vi "Grab Image.vi"() -> ()   [LabVIEW 2014]
uses:
  4.Other/header ctl/Offset.ctl
  4.Other/header ctl/file number.ctl
  <vilib>/vision/Image Controls.llb/IMAQ Image.ctl
  <vilib>/userdefined/High Color/IMAQdx.ctl
  4.Other/header ctl/Header file data.ctl
  4.Other/header ctl/Offset table.ctl
  <vilib>/Analysis/baseanly.llb/Mean (DBL).vi
  <vilib>/vision/driver/NI_Vision_Acquisition_Software.lvlib
  <resource>/objmgr/imaqdx.rc
  <vilib>/vision/NI_Vision_Development_Module.lvlib
  <vilib>/Analysis/NI_AALBase.lvlib
panel:
  in  "Reset BM":bool
  out "error out":errorcluster
  out "Global Rectangle":i32[](array[numeric])
  out "BMy array":dbl[](array[numeric])
  out "BMx array":dbl[](array[numeric])
  out "y array":dbl[](array[numeric])
  out "x array":dbl[](array[numeric])
  in  "AutoGain":enum16{"None", "Auto Once", "Continuous"}(ring)
  out "mean fps":dbl format="%0.2f"
  in  "Array":string[](array[string])=["BMx (nm)", "BMy (nm)", "xy ratio"]
  out "Results":dbl[](array[numeric])
  out "Saved Frame":u32
  out "acquire time array (ms)":u32[](array[numeric])
  in  "Extract bead?":bool
  out "frame acquired":i32
  out "Offset array":cluster{"offset":T1, "file number":T2}[](array[cluster])
  out "resized TTB":u32[](array[numeric])
  out "True acquired frame":u32
  in  "wait time between \neach grab (ms)":u32=30
  out "fps (Hz)":dbl
  out "TTB array (ms)\ntime axis (ms)":u32[](array[numeric])
  out "Glimpse refnum Array":refnum<file>[](array[refnum])
  in  "T = Stop Record":bool
  in  "T = Record Sequence":bool
  out "Finish Save?":bool
  out "Pixel depth":i16
  out "Path String Array":string[](array[string])
  in  "Tab Control":T3(tab)
  in  "Set Record Frame#":u32=30000
  out "Width":i32
  out "Height":i32
  in  "Data type":enum16{"U8", "I16"}(ring)
  in  "Select a Folder":path
  out "size of one frame (byte)":u32
  out "Frame# of one .Glimpse \n(2Gb)":u32
  out "Estimated total file size (byte, b)":u32
  out "Estimated total file size (Kb)":dbl
  out "image in Queue":i32(slide) min=0 max=180 step=30 scale=0.18..200.0
  out "pixel# of a image":i32
  out "Estimated a file size (byte, b)":u32
  out "Write to file num":u32
  out "avg. fps for recording (Hz)":dbl
  in  "Set Height":dbl=630.0
  in  "Set Width":dbl=1120.0
  in  "T = Auto-Set Exposure\nF = Manual":bool=TRUE
  in  "Manual Set\nExposure Time (ms)":dbl=30.0
  out "Image Display":T4(plugin-control)
  out "Image Extracted":T4(plugin-control)
  # "1120"
  # "width : max 1920"
  # "height max : 1200"
  # "630"
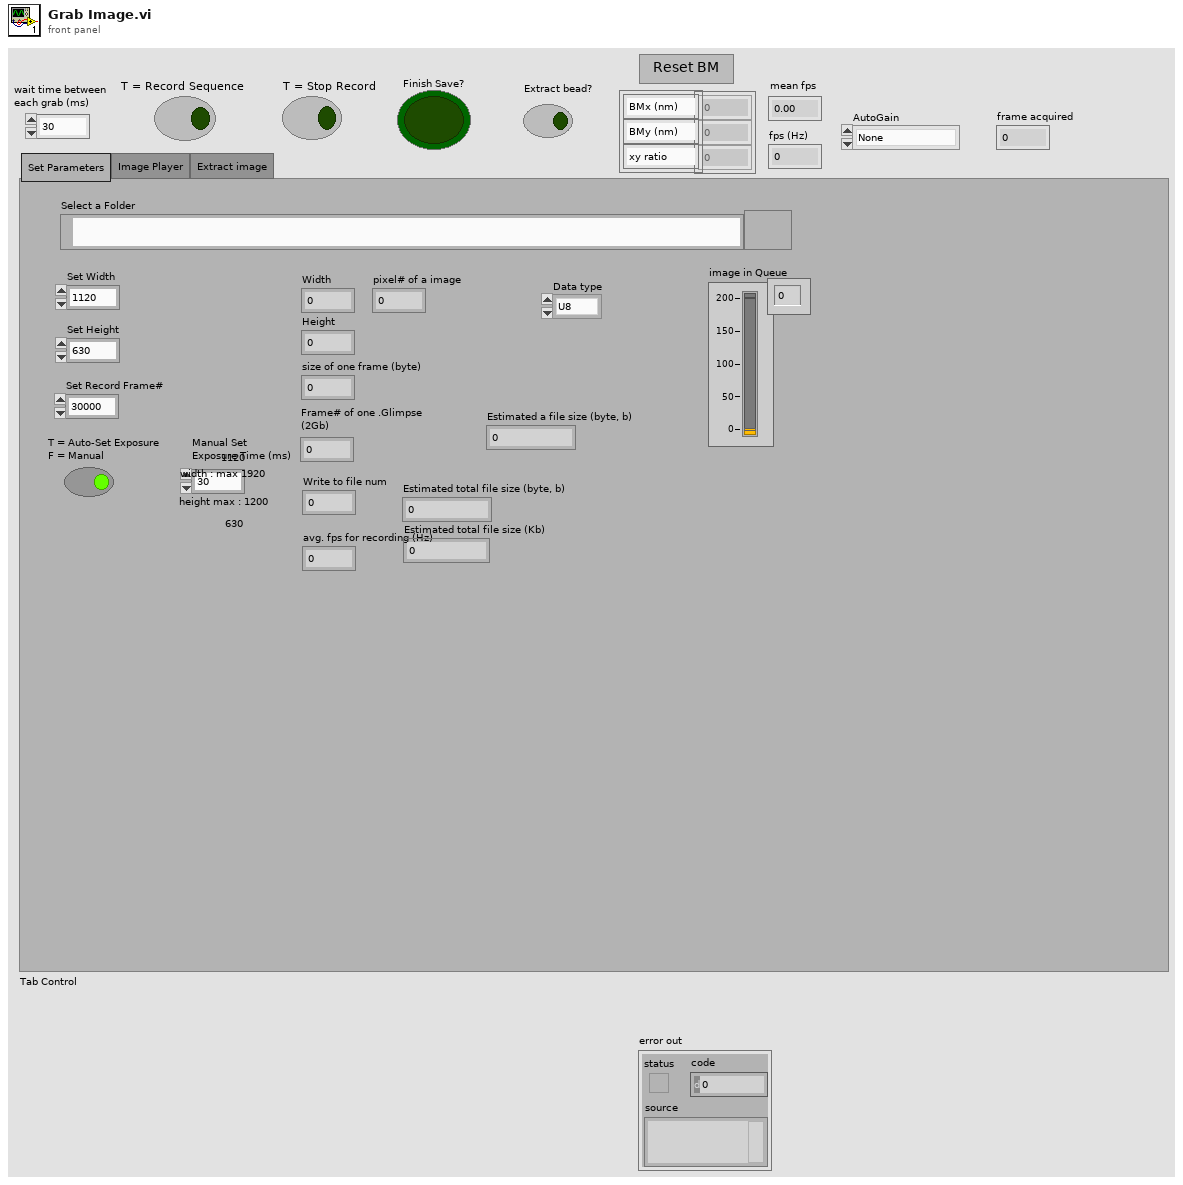
[diagram p1: front panel]
types:
  T1 = typedef "Offset.ctl" = i32
  T2 = typedef "file number.ctl" = u8
  T3 = enum32{"Set Parameters", "Image Player", "Extract image"}
  T4 = typedef "IMAQ Image.ctl" = refnum<image>
  T5 = typedef "IMAQdx.ctl" = refnum<k21>
  T6 = typedef "Image Type" = u32
  T7 = cluster{"Grab Image":T4, "max queue size (-1, unlimited)":u32}
  T8 = cluster{"Global Rectangle":i32[], "Contours":cluster{"Contour Type":u32, "ROI Type":u32, "Points":i32[]}[]}
  T9 = enum16{"open", "replace", "create", "open or create", "replace or create", "replace or create with confirmation"}
  T10 = typedef "Header file data.ctl" = cluster{"Frames Acquired":u32, "Region width":i32, "Region height":i32, "Element 0 of TTB":u32, "time of 1st frame, \nsec since 1/1/04":dbl, "TTB Array (ms)":u32[], "Offsets Array":T11, "Pixel depth":u32}
  T11 = typedef "Offset table.ctl" = cluster{"offset":T1, "file number":T2}[]
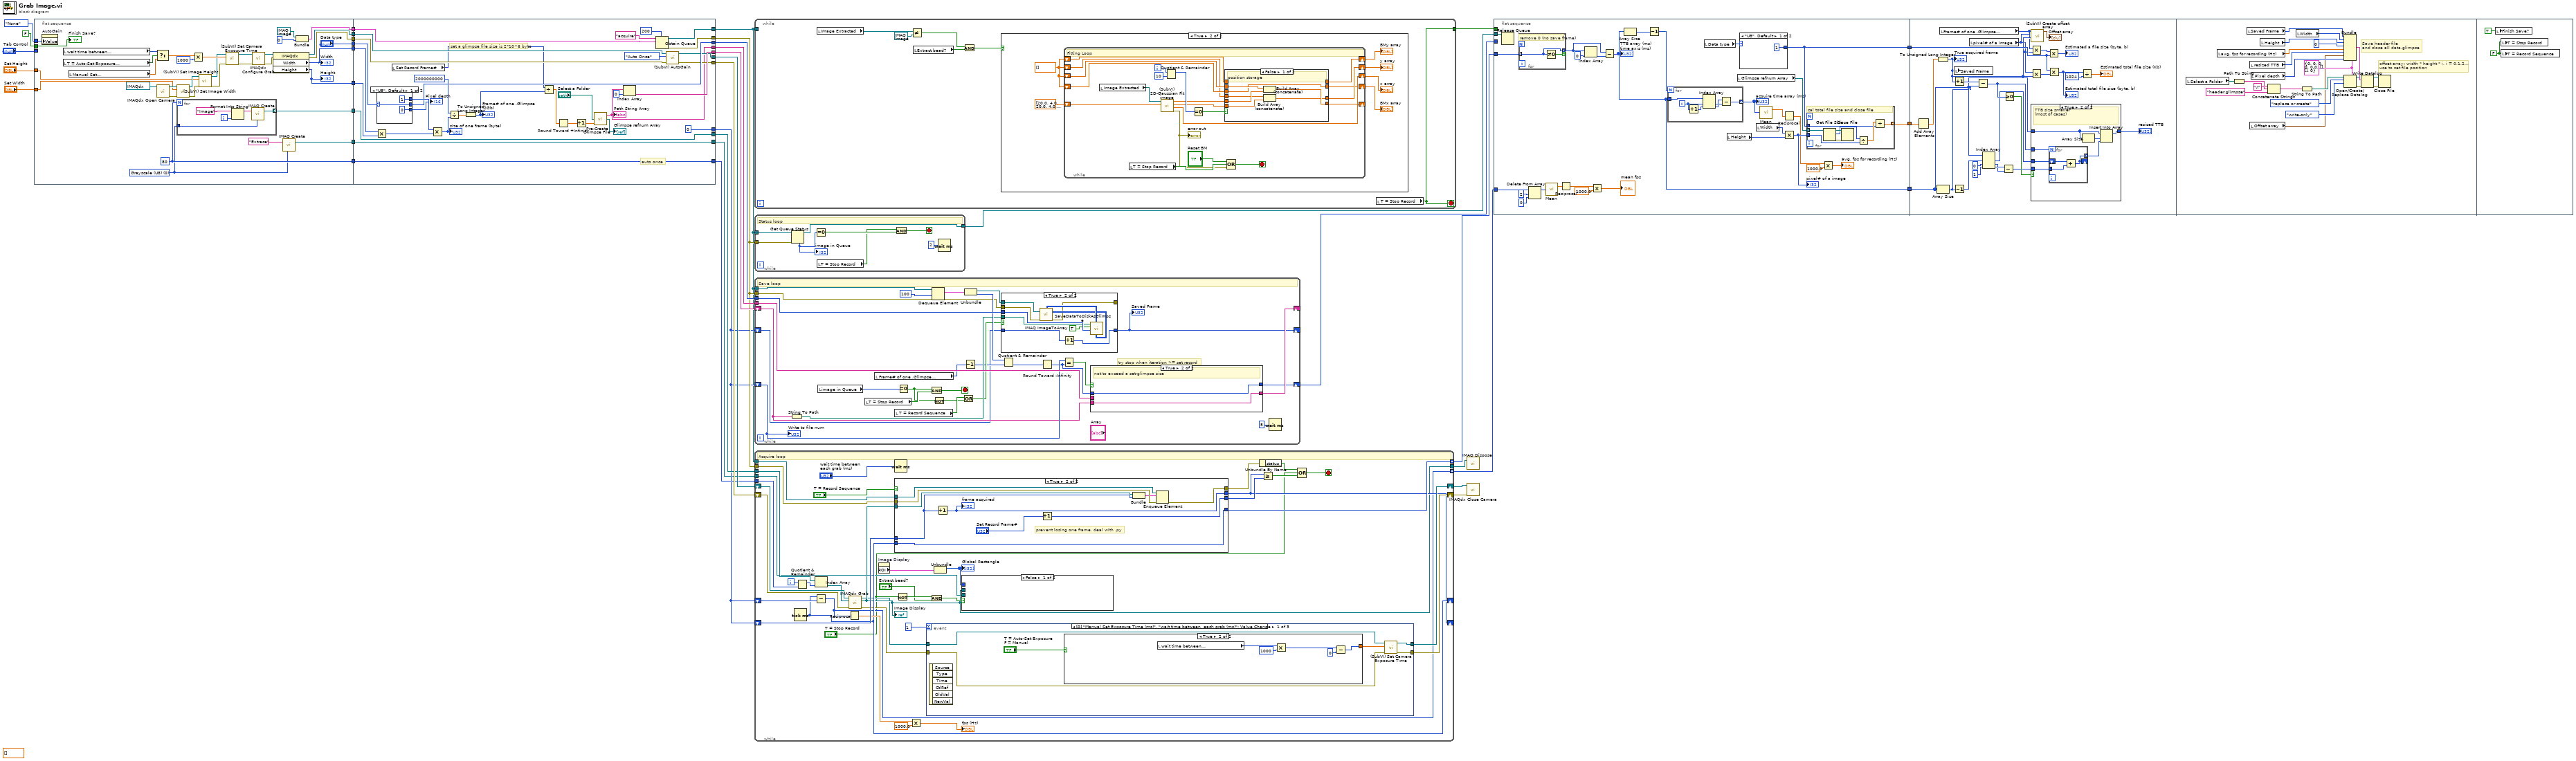
[diagram p0: block diagram]
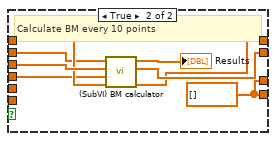
[diagram p3: hidden frame]
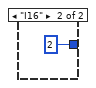
[diagram p4: hidden frame]
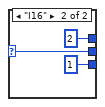
[diagram p6: hidden frame]
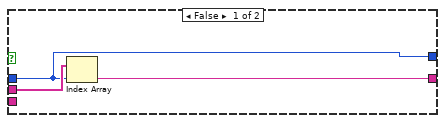
[diagram p8: hidden frame]
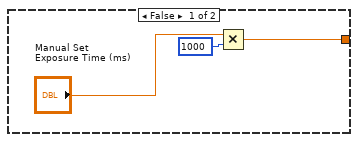
[diagram p9: hidden frame]
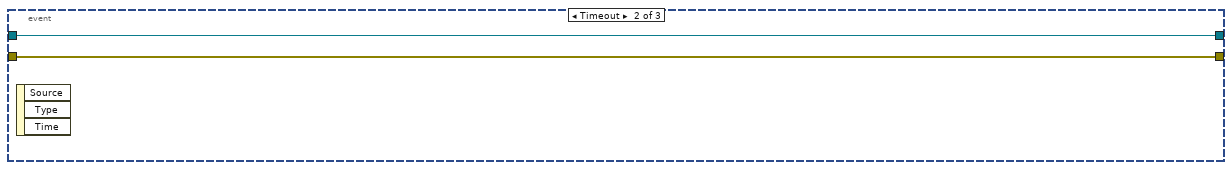
[diagram p10: hidden frame]
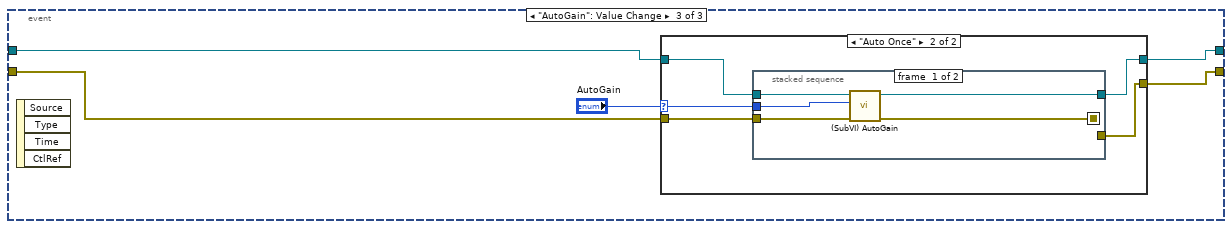
[diagram p11: hidden frame]
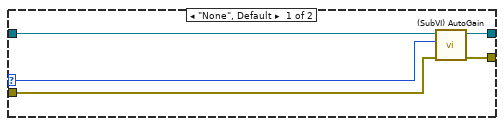
[diagram p12: hidden frame]
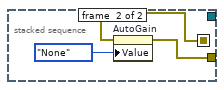
[diagram p13: hidden frame]
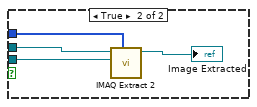
[diagram p14: hidden frame]
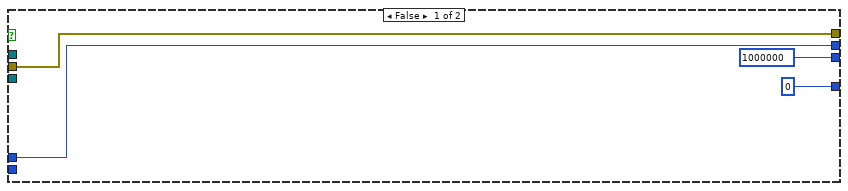
[diagram p15: hidden frame]
diagram:
  (unwired) dbl[] []
  n1 = flat-sequence {
    tunnel: [w61] -> w33
    tunnel: [w60] -> w32
    tunnel: [w70] -> w29
    tunnel: [w69] -> w28
    tunnel: ["Data type"] -> w26
    tunnel: [w65] -> w24
    tunnel: [w59] -> w21
    tunnel: [w58] -> w19
    tunnel: "Tab Control" -> [_]
    tunnel: FALSE ("Finish Save?") -> [w57]
    tunnel: "Set Width" -> [w43]
    tunnel: "Set Height" -> [w42]
    tunnel: [w54] -> w6
    tunnel: enum16{"None", "Auto Once", "Continuous"}."None" ("AutoGain") -> [w41]
    tunnel: [w88] -> w30
    tunnel: w33 -> [w90]
    tunnel: [w87] -> w31
    tunnel: w32 -> [w89]
    tunnel: w29 -> [w109]
    tunnel: w28 -> [w108]
    tunnel: w26 -> [w102]
    tunnel: [w101] -> w25
    tunnel: w24 -> [w95]
    tunnel: [w100] -> w20
    tunnel: w21 -> [w100]
    tunnel: [w99] -> w18
    tunnel: w19 -> [w99]
    tunnel: [w85] -> w16
    tunnel: [0] -> w10
    tunnel: [w96] -> w12
    tunnel: [w94] -> w2
    tunnel: [w93] -> w11
    tunnel: w6 -> [w77]
    tunnel: [w77] -> w5
    frame #0 {
      w58 = 80 ("# Of Buffers")
      w55 = T6 0 items=["Grayscale (U8)", "Grayscale (I16)", "Grayscale (SGL)", "Complex (CSG)", "RGB (U32)", "HSL (U32)", "RGB (U64)", "Grayscale (U16)"] ("Image Type")
      n2 = property on="AutoGain" class="Enum (strict)"("Value"=w41) -> ()  [unwired: 2 in, 2 out]
      n3 = local read "wait time between \neach grab (ms)"() -> (w38:u32)
      n4 = local read "T = Auto-Set Exposure\nF = Manual"() -> (w40:bool)
      n5 = local read "Manual Set\nExposure Time (ms)"() -> (w39:dbl)
      n6 = Select(t=w38, s=w40, f=w39) -> (s? t:f=w37:dbl)
      n7 = call <vilib>:"IMAQdx Open Camera.vi"("Session In"=T5 "cam2") -> ("error out"=w44:errorcluster, "Session Out"=w49:T5)  [unwired: 9 in]
      n8 = call "(SubVI) Set Image Width.vi"("error in (no error)"=w44, "Set Width"=w43, "Refnum in"=w49) -> ("error out"=w45:errorcluster, "Refnum out"=w48:T5)  [unwired: 7 in]
      n9 = for {
        N: w58 -> [_]
        tunnel: [w75] -> w59 mode=indexing
        tunnel: w55 -> [w71]
        i -> [w74]
        n10 = Format Into String(initial string="Image" ("Image Name"), w74) -> (resulting string=w72:string)  [unwired: 2 in, 1 out]
        n11 = call "IMAQ Create"("Image Name"=w72, "Image Type"=w71) -> ("New Image"=w75:T4)  [unwired: 3 in, 1 out]
      }
      n12 = Multiply(x=w37, y=u32 1000) -> (x*y=w50:dbl)
      n13 = call "(SubVI) Set Image Height.vi"("error in (no error)"=w45, "Set Height"=w42, "Refnum in"=w48) -> ("error out"=w46:errorcluster, "Refnum out"=w47:T5)  [unwired: 7 in]
      n14 = call "(SubVI) Set Camera Exposure Time.vi"("error in (no error)"=w46, "ExposureTime (us)"=w50, "Refnum in"=w47) -> ("error out"=w53:errorcluster, "Refnum out"=w52:T5)  [unwired: 7 in]
      n15 = call <vilib>:"IMAQdx Configure Grab.vi"("error in"=w53, "Session In"=w52) -> ("error out"=w62:errorcluster, "Session Out"=w63:T5)  [unwired: 8 out]
      n16 = property class="IMAQdx"(reference=w63, error in=w62) -> (reference out=w61:T5, error out=w60:errorcluster, "Width"=w70:u32, "Height"=w69:u32)
      "Width" <- w70
      "Height" <- w69
      n17 = call "IMAQ Create"("Image Name"="Extrace", "Image Type"=w55) -> ("New Image"=w54:T4)  [unwired: 3 in, 1 out]
      n18 = Bundle("Grab Image"=T4 refnum, "max queue size (-1, unlimited)"=u32 0) -> (w65:T7)  [unwired: 1 in]
      "Finish Save?" <- w57
    }
    frame #1 {
      # "auto once"
      # "set a glimpse file size is 2*10^6 byte"
      n19 = Multiply(x=w109, y=w108) -> (x*y=w107:u32)
      n20 = case shown="\"U8\", Default" w102 {
        selector: w102 -> [w111 w114]
        tunnel: [1 2] -> w106
        tunnel: [w111 w114] -> w101
        tunnel: [i16 0 i16 1] -> w91
        frame "U8", Default {
        }
        frame "I16" {
        }
      }
      "Pixel depth" <- w91
      n21 = local read "Set Record Frame#"() -> (w83:u32)
      n22 = Multiply(x=w106, y=w107) -> (x*y=w104:u32)
      "size of one frame (byte)" <- w104
      n23 = Divide(x=2000000000, y=w104) -> (x/y=w103:dbl)
      n24 = To Unsigned Long Integer(number=w103) -> (unsigned 32bit integer=w82:u32)
      "Frame# of one .Glimpse \n(2Gb)" <- w82
      n25 = Divide(x=w83, y=w82) -> (x/y=w81:dbl)
      n26 = Round Toward +Infinity(x=w81) -> (ceil(x): smallest int >= x=w80:dbl)
      n27 = Increment(x=w80) -> (x+1=w79:dbl)
      n28 = call "Pre-Create Glimpse File.vi"("pre-created file #"=w79, "Select a Folder"="Select a Folder") -> ("refnum Array"=→"Glimpse refnum Array":refnum<file>[], "Path String Array"=w85:string[])  [unwired: 2 in]
      "Path String Array" <- w85
      n29 = Index Array(array=w85, index=0) -> (element=w96:string)
      n30 = Obtain Queue(max queue size (-1, unlimited)=200, name (unnamed)="acquire", element data type=w95) -> (queue out=w94:refnum<queue>, error out=w93:errorcluster)  [unwired: 2 in, 1 out]
      n31 = call "(SubVI) AutoGain.vi"("error in (no error)"=w89, "AutoMode"=enum16{"None", "Auto Once", "Continuous"}."Auto Once", "Refnum in"=w90) -> ("error out"=w87:errorcluster, "Refnum out"=w88:T5)  [unwired: 7 in]
    }
  }
  n32 = while {
    tunnel: w2 -> [_]
    tunnel: [w119] -> w1
    stop <- w119 stop-if-true
    n33 = local read "Image Extracted"() -> (w121:T4)
    n34 = Not Equal?(x=w121, y=T4 refnum ("Grab Image")) -> (x != y?=w118:bool)
    n35 = local read "Extract bead?"() -> (w117:bool)
    n36 = And(x=w118, y=w117) -> (x .and. y?=w116:bool)
    n37 = case shown="True" w116 {
      frame False {
      }
      frame True {
        w127 = dbl[] []
        n38 = while {
          shift-right: [w133] -> w126
          shift-left: w127 -> [w142]
          shift-right: [w132] -> w125
          shift-left: w127 -> [w141]
          shift-right: [w134] -> w124
          shift-left: w127 -> [w140]
          shift-right: [w135] -> w123
          shift-left: w127 -> [w139]
          shift-right: [w138] -> _
          shift-left: dbl[] [20.0, 4.0, 20.0, 4.0, 40.0, 127.0] ("initial parameters") -> [w137]
          i -> [w143]
          stop <- w128 stop-if-true
          # "Fitting Loop"
          n39 = local read "Image Extracted"() -> (w136:T4)
          n40 = local read "T = Stop Record"() -> (w130:bool)
          n41 = call "(SubVI) 2D-Gaussian Fit image.vi"("initial parameters"=w137, "Input Image"=w136) -> ("error out"=w129:errorcluster, "best fit parameters"=w138:dbl[], "y position (nm)"=w145:dbl, "x position (nm)"=w146:dbl)  [unwired: 6 in]
          "error out" <- w129
          n42 = Quotient & Remainder(x=w143, y=10) -> (x-y*floor(x/y)=w147:i32)  [unwired: 1 out]
          n43 = Equal To 0?(x=w147) -> (x = 0?=w144:bool)
          n44 = case shown="False" w144 {
            tunnel: w142 -> [w153 w159]
            tunnel: w140 -> [w152 w158]
            tunnel: [w154 w160] -> w133
            tunnel: [w151 w160] -> w134
            tunnel: [w150 w164] -> w132
            tunnel: [w149 w163] -> w135
            tunnel: w141 -> [w150 w162]
            tunnel: w139 -> [w149 w161]
            tunnel: w146 -> [w156 _]
            tunnel: w145 -> [w155 _]
            frame False {
              # "position storage"
              n45 = Build Array (concatenate)(w153, w156) -> (w154:dbl[])
              n46 = Build Array (concatenate)(w152, w155) -> (w151:dbl[])
            }
            frame True {
              w160 = dbl[] []
              # "Calculate BM every 10 points"
              n47 = call "(SubVI) BM calculator.vi"("BMy array in (nm)"=w161, "y position array in (nm)"=w158, "BMx array in (nm)"=w162, "x position array in (nm)"=w159) -> ("BMy array appended (nm)"=w163:dbl[], "BMx array appended (nm)"=w164:dbl[], "Results"=→"Results":dbl[])  [unwired: 1 in]
            }
          }
          n48 = Compound Arithmetic op=OR("Reset BM", w130, w129) -> (w128:bool)
        }
        "x array" <- w126
        "y array" <- w124
        "BMx array" <- w125
        "BMy array" <- w123
      }
    }
    n49 = local read "T = Stop Record"() -> (w119:bool)
  }
  n50 = while {
    tunnel: w2 -> [w172]
    tunnel: [w171] -> w22
    tunnel: w11 -> [w170]
    stop <- w165 stop-if-true
    # "Status loop"
    n51 = Get Queue Status(queue=w172, error in (no error)=w170) -> (queue out=w171:refnum<queue>, # elements in queue=w168:i32)  [unwired: 1 in, 6 out]
    "image in Queue" <- w168
    n52 = Equal To 0?(x=w168) -> (x = 0?=w169:bool)
    n53 = local read "T = Stop Record"() -> (w166:bool)
    n54 = And(x=w166, y=w169) -> (x .and. y?=w165:bool)
    n55 = Wait (ms)(milliseconds to wait=u32 2) -> ()  [unwired: 1 out]
  }
  n56 = while {
    tunnel: w2 -> [w201]
    tunnel: w11 -> [w200]
    tunnel: w25 -> [w199]
    shift-right: [w188] -> w23
    shift-left: w10 -> [w193]
    shift-right: [w192] -> _
    shift-left: w12 -> [w190]
    tunnel: w16 -> [w194]
    shift-right: [w173] -> _
    shift-left: w10 -> [w174]
    stop <- w177 stop-if-true
    # "try stop when iteration >= set record"
    # "Save loop"
    n57 = String To Path(string=w190) -> (path=w191:path)
    n58 = local read "image in Queue"() -> (w183:i32)
    n59 = local read "T = Stop Record"() -> (w185:bool)
    n60 = local read "Frame# of one .Glimpse \n(2Gb)"() -> (w175:u32)
    n61 = local read "T = Record Sequence"() -> (w182:bool)
    n62 = Equal To 0?(x=w183) -> (x = 0?=w180:bool)
    n63 = And(x=w180, y=w185) -> (x .and. y?=w177:bool)
    n64 = Dequeue Element(queue=w201, timeout in ms (-1)=100, error in (no error)=w200) -> (element=w198:T7, error out=w184:errorcluster)  [unwired: 2 out]
    n65 = Not(x=w180) -> (.not. x?=w181:bool)
    n66 = Or(x=w182, y=w181) -> (x .or. y?=w179:bool)
    n67 = Decrement(x=w175) -> (x-1=w176:u32)
    n68 = Unbundle(w198) -> ("Grab Image"=w187:T4, "max queue size (-1, unlimited)"=w197:u32)
    n69 = case shown="True" w179 {
      tunnel: w199 -> [_ w213]
      tunnel: w191 -> [_ w212]
      tunnel: w187 -> [_ w208]
      tunnel: w184 -> [w203 w207]
      tunnel: [w203 w206] -> _
      tunnel: w174 -> [w202 w205]
      tunnel: [w202 w204] -> w173
      frame False {
      }
      frame True {
        n70 = call "IMAQ ImageToArray"("error in (no error)"=w207, "Image"=w208) -> ("error out"=w206:errorcluster, "Image Pixels (U8)"=w210:u8[][], "Image Pixels (I16)"=w209:i16[][])  [unwired: 2 in, 2 out]
        n71 = Increment(x=w205) -> (x+1=w204:i32)
        n72 = call "SaveDataToDiskAsGlimpse.vi"("Read or Write Path"=w212, "Array (U8)"=w210, "T = AddNewData\nF = if exist, OverWrite or CreateNew"=TRUE ("T = AddNewData\nF = if exist, OverWrite or CreateNew"), "Data type"=w213, "Array (I16)"=w209) -> ()  [unwired: 3 in, 1 out]
      }
    }
    "Saved Frame" <- w173
    n73 = Quotient & Remainder(x=w197, y=w176) -> (floor(x/y)=w196:u32)  [unwired: 1 out]
    n74 = Round Toward -Infinity(1:w196) -> (0:w189:u32)
    n75 = Equal?(x=w193, y=w189) -> (x = y?=w195:bool)
    n76 = case shown="True" w195 {
      tunnel: w194 -> [w216 _]
      tunnel: w189 -> [w214 w217]
      tunnel: [w215 w218] -> w192
      tunnel: w190 -> [_ w218]
      tunnel: [w214 w217] -> w188
      frame False {
        n77 = Index Array(array=w216, index=w214) -> (element=w215:string)
      }
      frame True {
        # "not to exceed a set-glimpse size"
      }
    }
    n78 = Wait (ms)(milliseconds to wait=u32 5) -> ()  [unwired: 1 out]
    "Write to file num" <- w193
  }
  n79 = while {
    tunnel: [w231] -> w34
    tunnel: w2 -> [w253]
    shift-right: [w233] -> _
    shift-left: w10 -> [w249]
    tunnel: w11 -> [w248]
    shift-right: [w235] -> _
    shift-left: w10 -> [w247]
    tunnel: w20 -> [w242]
    tunnel: w18 -> [w240]
    tunnel: [w234] -> w17 mode=indexing
    shift-right: [w236] -> w36
    shift-left: w30 -> [w256]
    shift-right: [w237] -> w35
    shift-left: w31 -> [w255]
    tunnel: w5 -> [w232]
    tunnel: [w226] -> w4 mode=indexing
    i -> [w225]
    stop <- w238 stop-if-true
    # "Acquire loop"
    n80 = Tick Count (ms)() -> (millisecond timer value=w235:u32)
    n81 = Quotient & Remainder(x=w225, y=w240) -> (x-y*floor(x/y)=w243:i32)  [unwired: 1 out]
    n82 = Subtract(x=w235, y=w247) -> (x-y=w226:u32)
    n83 = Index Array(array=w242, index=w243) -> (element=w241:T4)
    n84 = Reciprocal(x=w226) -> (1/x=w246:dbl)
    n85 = call <vilib>:"IMAQdx Grab.vi"("error in"=w255, "Image In"=w241, "Session In"=w256) -> ("error out"=w228:errorcluster, "Image Out"=w231:T4, "Session Out"=w229:T5)  [unwired: 1 in, 5 out]
    "Image Display" <- w231
    n86 = property on="Image Display" class="ImageControl"() -> ("ROI"=w230:T8)  [unwired: 2 in, 2 out]
    n87 = Wait (ms)(milliseconds to wait="wait time between \neach grab (ms)") -> ()  [unwired: 1 out]
    n88 = case shown="True" "T = Record Sequence" {
      tunnel: w253 -> [_ w313]
      tunnel: w231 -> [_ w310]
      tunnel: w248 -> [w303 w312]
      tunnel: [w303 w311] -> w252
      tunnel: w249 -> [w302 w309]
      tunnel: [w302 w308] -> w233
      tunnel: [u32 1000000 ("Set Record Frame#") w304] -> w239
      tunnel: [u32 0 ("millisecond timer value") w306] -> w234
      tunnel: w235 -> [_ w306]
      frame False {
      }
      frame True {
        # "prevent losing one frame, deal with .py"
        n89 = Increment(x=w309) -> (x+1=w308:i32)
        "frame acquired" <- w308
        n90 = Increment(x="Set Record Frame#") -> (x+1=w304:u32)
        n91 = Bundle("Image Out"=w310, w309) -> (w307:cluster{"Image Out":T4, i32})  [unwired: 1 in]
        n92 = Enqueue Element(queue=w313, element=w307, error in (no error)=w312) -> (error out=w311:errorcluster)  [unwired: 1 in, 2 out]
      }
    }
    n93 = Not(x="T = Stop Record") -> (.not. x?=w222:bool)
    n94 = Multiply(x=w246, y=1000.0) -> (x*y=→"fps (Hz)":dbl)
    n95 = event shown="[0] \"Manual Set Exposure Time (ms)\", \"wait time between  each grab (ms)\": Value Change" {
      selector: _ -> [_ _ _]
      dyn-events: _ -> [_ _ _]
      timeout: 1 -> [_ _ _]
      tunnel: w229 -> [w262 w272 w277]
      tunnel: [w261 w272 w275] -> w236
      tunnel: w228 -> [w260 w271 w276]
      tunnel: [w259 w271 w273] -> w237
      event "Manual Set\nExposure Time (ms)", "wait time between \neach grab (ms)": Value Change {
        n96 = event-data() -> ()  [unwired: 1 in, 6 out]
        n97 = case shown="True" "T = Auto-Set Exposure\nF = Manual" {
          tunnel: [w263 w267] -> w257
          frame False {
            n98 = Multiply(x="Manual Set\nExposure Time (ms)", y=u32 1000) -> (x*y=w263:dbl)
          }
          frame True {
            n99 = local read "wait time between \neach grab (ms)"() -> (w266:u32)
            n100 = Multiply(x=w266, y=u32 1000) -> (x*y=w269:u32)
            n101 = Subtract(x=w269, y=u32 0) -> (x-y=w267:u32)
          }
        }
        n102 = call "(SubVI) Set Camera Exposure Time.vi"("error in (no error)"=w260, "ExposureTime (us)"=w257, "Refnum in"=w262) -> ("error out"=w259:errorcluster, "Refnum out"=w261:T5)  [unwired: 7 in]
      }
      event Timeout {
        n103 = event-data() -> ()  [unwired: 1 in, 3 out]
      }
      event "AutoGain": Value Change {
        n104 = event-data() -> ()  [unwired: 1 in, 4 out]
        n105 = case shown="\"Auto Once\"" "AutoGain" {
          selector: "AutoGain" -> [w282 w283]
          tunnel: w277 -> [w281 w287]
          tunnel: w276 -> [w279 w286]
          tunnel: [w280 w285] -> w275
          tunnel: [w278 w284] -> w273
          frame "None", Default {
            n106 = call "(SubVI) AutoGain.vi"("error in (no error)"=w279, "AutoMode"=w282, "Refnum in"=w281) -> ("error out"=w278:errorcluster, "Refnum out"=w280:T5)  [unwired: 7 in]
          }
          frame "Auto Once" {
            n107 = stacked-sequence {
              seq-local: [w289 _] -> [_ w294]
              tunnel: w287 -> [w292 _]
              tunnel: w286 -> [w291 _]
              tunnel: [w290 _] -> w285
              tunnel: [_ w293] -> w284
              tunnel: w283 -> [w288 _]
              frame #0 {
                n108 = call "(SubVI) AutoGain.vi"("error in (no error)"=w291, "AutoMode"=w288, "Refnum in"=w292) -> ("error out"=w289:errorcluster, "Refnum out"=w290:T5)  [unwired: 7 in]
              }
              frame #1 {
                n109 = property on="AutoGain" class="Enum (strict)"(error in=w294, "Value"=enum16{"None", "Auto Once", "Continuous"}."None" ("AutoGain")) -> (error out=w293:errorcluster)  [unwired: 1 in, 1 out]
              }
            }
          }
        }
      }
    }
    n110 = And(x=w222, y="Extract bead?") -> (x .and. y?=w220:bool)
    n111 = Unbundle(w230) -> ("Global Rectangle"=w219:i32[])  [unwired: 1 out]
    "Global Rectangle" <- w219
    n112 = case shown="False" w220 {
      tunnel: w219 -> [_ w299]
      tunnel: w232 -> [_ w298]
      tunnel: w231 -> [_ w297]
      frame False {
      }
      frame True {
        n113 = call "IMAQ Extract 2"("Optional Rectangle"=w299, "Image Dst"=w298, "Image Src"=w297) -> ("Image Dst Out"=→"Image Extracted":T4)  [unwired: 7 in, 1 out]
      }
    }
    n114 = Unbundle By Name(w252) -> ("status"=w254:bool)
    n115 = Greater Or Equal?(x=w233, y=w239) -> (x >= y?=w251:bool)
    n116 = Compound Arithmetic op=OR(w254, "T = Stop Record", w251) -> (w238:bool)
  }
  n117 = call "IMAQ Dispose"("Image"=w34) -> ()  [unwired: 5 in, 1 out]
  n118 = call <vilib>:"IMAQdx Close Camera.vi"("error in"=w35, "Session In"=w36) -> ()  [unwired: 10 out]
  n119 = flat-sequence {
    tunnel: w23 -> [_]
    tunnel: w17 -> [w331]
    tunnel: w22 -> [w340]
    tunnel: [w333] -> w15
    tunnel: [w327] -> w14
    tunnel: [w332] -> w13
    tunnel: w4 -> [w321]
    tunnel: w1 -> [_]
    tunnel: w15 -> [w381]
    tunnel: w14 -> [w370]
    tunnel: w13 -> [w366]
    frame #0 {
      n120 = Release Queue(queue=w340) -> ()  [unwired: 1 in, 4 out]
      n121 = for {
        tunnel: w331 -> [w349] mode=indexing
        tunnel: [w349] -> w330 mode=indexing if=w348
        # "remove 0 (no save frame)"
        n122 = Not Equal To 0?(x=w349) -> (x != 0?=w348:bool)
      }
      n123 = Delete From Array(array=w321, length=2, index=0) -> (array with subset deleted=w318:u32[])  [unwired: 1 out]
      n124 = call-poly <vilib>:"Mean.vi"("X"=w318) -> ("mean"=w317:dbl)  [unwired: 1 out]
      n125 = Reciprocal(x=w317) -> (1/x=w316:dbl)
      n126 = Index Array(array=w330, index=0) -> (element=w337:u32)
      n127 = Multiply(x=w316, y=1000.0) -> (x*y=→"mean fps":dbl)
      n128 = Subtract(x=w330, y=w337) -> (x-y=w327:u32[])
      "TTB array (ms)\ntime axis (ms)" <- w327
      n129 = Array Size(array=w327) -> (size(s)=w329:i32)
      n130 = Decrement(x=w329) -> (x-1=w328:i32)
      n131 = for {
        N: w328 -> [_]
        tunnel: w327 -> [w347]
        tunnel: [w342] -> w322 mode=indexing
        i -> [w346]
        n132 = Increment(x=w346) -> (x+1=w345:i32)
        n133 = Index Array(array=w347, index #1=w346, index #2=w345) -> (element #1=w343:u32, element #2=w344:u32)
        n134 = Subtract(x=w344, y=w343) -> (x-y=w342:u32)
      }
      "acquire time array (ms)" <- w322
      n135 = local read "Data type"() -> (w335:enum16{"U8", "I16"})
      n136 = local read "Height"() -> (w338:i32)
      n137 = local read "Glimpse refnum Array"() -> (w341:refnum<file>[])
      n138 = case shown="\"U8\", Default" w335 {
        tunnel: [1 2] -> w332
        frame "U8", Default {
        }
        frame "I16" {
        }
      }
      n139 = local read "Width"() -> (w339:i32)
      n140 = call-poly <vilib>:"Mean.vi"("X"=w322) -> ("mean"=w326:dbl)  [unwired: 1 out]
      n141 = Reciprocal(x=w326) -> (1/x=w325:dbl)
      n142 = Multiply(x=w339, y=w338) -> (x*y=w334:i32)
      "pixel# of a image" <- w334
      n143 = for {
        tunnel: w341 -> [w359] mode=indexing
        tunnel: w334 -> [w355]
        tunnel: [w352] -> w333 mode=indexing
        tunnel: w332 -> [w353]
        # "cal total file size and close file"
        n144 = Get File Size(file=w359) -> (refnum out=w358:refnum<file>, size (in bytes)=w356:i64, 0:w357:errorcluster)  [unwired: 1 in]
        n145 = Close File(refnum=w358, error in=w357) -> ()  [unwired: 2 out]
        n146 = Divide(x=w356, y=w355) -> (x/y=w354:dbl)
        n147 = Divide(x=w354, y=w353) -> (x/y=w352:dbl)
      }
      n148 = Multiply(x=w325, y=1000.0) -> (x*y=→"avg. fps for recording (Hz)":dbl)
    }
    frame #1 {
      n149 = Add Array Elements(numeric array=w381) -> (sum=w380:dbl)
      n150 = To Unsigned Long Integer(number=w380) -> (unsigned 32bit integer=w363:u32)
      "True acquired frame" <- w363
      n151 = Array Size(array=w370) -> (size(s)=w368:i32)
      n152 = local read "Frame# of one .Glimpse \n(2Gb)"() -> (w362:u32)
      n153 = Increment(x=w363) -> (x+1=w375:u32)
      n154 = Decrement(x=w368) -> (x-1=w367:i32)
      n155 = local write "Saved Frame"(w363) -> ()
      n156 = local read "pixel# of a image"() -> (w361:i32)
      n157 = Subtract(x=w375, y=w368) -> (x-y=w373:u32)
      n158 = Index Array(array=w370, index #1=w367, index #2=0 ("index"), index #3=1 ("index")) -> (element #1=w372:u32, element #2=w384:u32, element #3=w385:u32)
      n159 = Subtract(x=w385, y=w384) -> (x-y=w371:u32)
      n160 = Greater Or Equal To 0?(x=w373) -> (x >= 0?=w374:bool)
      n161 = Multiply(x=w362, y=w361) -> (x*y=w365:u32)
      n162 = Multiply(x=w361, y=w363) -> (x*y=w376:u32)
      n163 = call "(SubVI) Create offset array.vi"("Frame #"=w363, "pixel# of a image"=w361, "Frame# of one .Glimpse \n(2Gb)"=w362) -> ("Array"=→"Offset array":cluster{"offset":T1, u32}[])  [unwired: 8 in]
      n164 = case shown="True" w374 {
        tunnel: w373 -> [_ w393]
        tunnel: w372 -> [_ w392]
        tunnel: w371 -> [_ w391]
        tunnel: w370 -> [w386 w389]
        tunnel: [w386 w388] -> w369
        frame False {
          # "TTB size always >= acquired frame"
        }
        frame True {
          # "TTB size smaller \n(most of cases)"
          n165 = for {
            N: w393 -> [_]
            tunnel: w391 -> [w395]
            shift-right: [w394] -> _
            shift-left: w392 -> [w396]
            tunnel: [w394] -> w390 mode=indexing
            n166 = Add(x=w396, y=w395) -> (x+y=w394:u32)
          }
          n167 = Array Size(array=w389) -> (size(s)=w387:i32)
          n168 = Insert Into Array(array=w389, index=w387, new element=w390) -> (w388:u32[])
        }
      }
      "resized TTB" <- w369
      n169 = Multiply(x=w365, y=w366) -> (x*y=→"Estimated a file size (byte, b)":u32)
      n170 = Multiply(x=w366, y=w376) -> (x*y=w377:u32)
      "Estimated total file size (byte, b)" <- w377
      n171 = Divide(x=w377, y=u32 1024) -> (x/y=→"Estimated total file size (Kb)":dbl)
    }
    frame #2 {
      w413 = T10 {"Frames Acquired"=0, "Region width"=0, "Region height"=0, "Element 0 of TTB"=0, "time of 1st frame, \nsec since 1/1/04"=0.0, "TTB Array (ms)"=[], "Offsets Array"=[], "Pixel depth"=0} ("Header file data")
      # "offset array: width * height * i, i = 0,1,2...\nuse to set file position"
      # "Save header file\nand close all data.glimpse"
      n172 = local read "Select a Folder"() -> (w407:path)
      n173 = local read "avg. fps for recording (Hz)"() -> (w397:dbl)
      n174 = Path To String(path=w407) -> (string=w405:string)
      n175 = local read "Saved Frame"() -> (w408:u32)
      n176 = local read "resized TTB"() -> (w399:u32[])
      n177 = local read "Offset array"() -> (w398:cluster{"offset":T1, "file number":T2}[])
      n178 = local read "Pixel depth"() -> (w412:i16)
      n179 = local read "Height"() -> (w410:i32)
      n180 = Concatenate Strings(w405, "\\" ("string"), "header.glimpse" ("string")) -> (w404:string)
      n181 = local read "Width"() -> (w409:i32)
      n182 = String To Path(string=w404) -> (path=w402:path)
      n183 = Bundle(cluster=w413, "Frames Acquired"=w408, "Region width"=w409, "Region height"=w410, "Element 0 of TTB"=u32 0, "time of 1st frame, \nsec since 1/1/04"=w397, "TTB Array (ms)"=w399, "Offsets Array"=w398, "Pixel depth"=w412) -> (w418:T10)
      n184 = Open/Create/Replace Datalog(5:w413, 9:enum16{"read/write", "read-only", "write-only"}."write-only" ("access (0:read/write)"), 10:T9."replace or create" ("operation (0:open)"), 11:w402) -> (0:w416:errorcluster, 3:w414:refnum<k1>)  [unwired: 1 in, 2 out]
      n185 = Write Datalog(4:w416, 6:w418, 7:w414) -> (0:w417:errorcluster, 3:w415:refnum<k1>)
      n186 = Close File(refnum=w415, error in=w417) -> ()  [unwired: 2 out]
    }
    frame #3 {
      w419 = FALSE
      n187 = local write "Finish Save?"(TRUE) -> ()
      n188 = local write "T = Stop Record"(w419) -> ()
      n189 = local write "T = Record Sequence"(w419) -> ()
    }
  }
